vi "main_state.vi"() -> ()   [LabVIEW 2012]
uses:
  machine_type.ctl
  <vilib>/LabVIEW Interface for Arduino/LabVIEW Interface for Arduino.lvlib
  LIFA Ultrasonic Distance LV9/LIFA Ultrasonic Distance.lvlib
  LIFA Ultrasonic Distance LV9/Get Distance/HC-SR04 Get Distance.vi
panel:
  in  "stop":bool
  in  "Plot Color":u32(colorbox)=16715776
  in  "Grid Color":u32(colorbox)
  in  "Visible Section":u16(ring)=8
  in  "Lines/Points":enum16{"Lines", "Points"}(ring)
  out "Polar Plot":picture
  out "Current angle (Degrees)":u8=15
  in  "Speed":u8=1
  in  "Servo 0 Sweep Max Angle":u8=180
  out "Current distance (cm)":dbl
  in  "Signal Pin":u8
  in  "Trigger Pin":u8
  in  "Servo Data Pin":u8=12
  in  "VISA resource":refnum<visa-resource-name>
  in  "Enum":T1
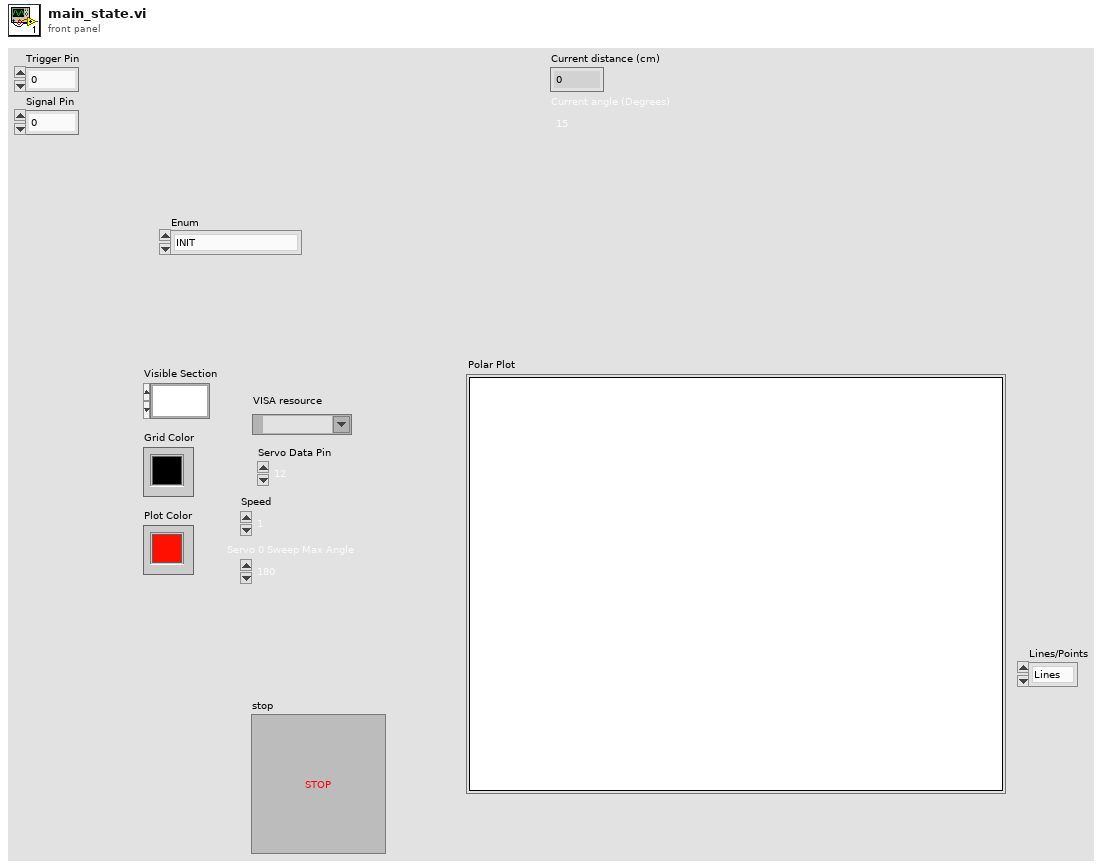
[diagram p1: front panel]
types:
  T1 = typedef "machine_type.ctl" = enum16{"INIT", "MEASURE_DIST", "MOVE_SERVO", "CLOSE", "PLOT_DATA", "ERROR"}
  T2 = typedef "LabVIEW Interface for Arduino.lvlib/Arduino Resource.ctl" = cluster{"VISA resource":refnum<visa-resource-name>, "Board Type":T3, "Connection Type":enum8{"USB / Serial"}, "Bytes Per Packet (15)":u8}
  T3 = typedef "LabVIEW Interface for Arduino.lvlib/Board Type.ctl" = enum16{"Uno", "Dimuelanove w/Atmega 328", "Mega 2560"}
  T4 = cluster{"maximum":dbl, "minimum":dbl, "clip to min":bool, "log?(F)":bool, "grid color":u32, "plot color":u32, "format and precision":cluster{"format":enum8{"Decimal", "Scientific", "Engineering", "Binary", "Octal", "Hex"}, "precision":u8}, "visible section":u16}
  T5 = typedef "LVBoundsTypeDef.ctl" = cluster{"Width":u32, "Height":u32}
  T6 = cluster{"Distance (cm)":dbl, "Angle (Degrees)":u8}
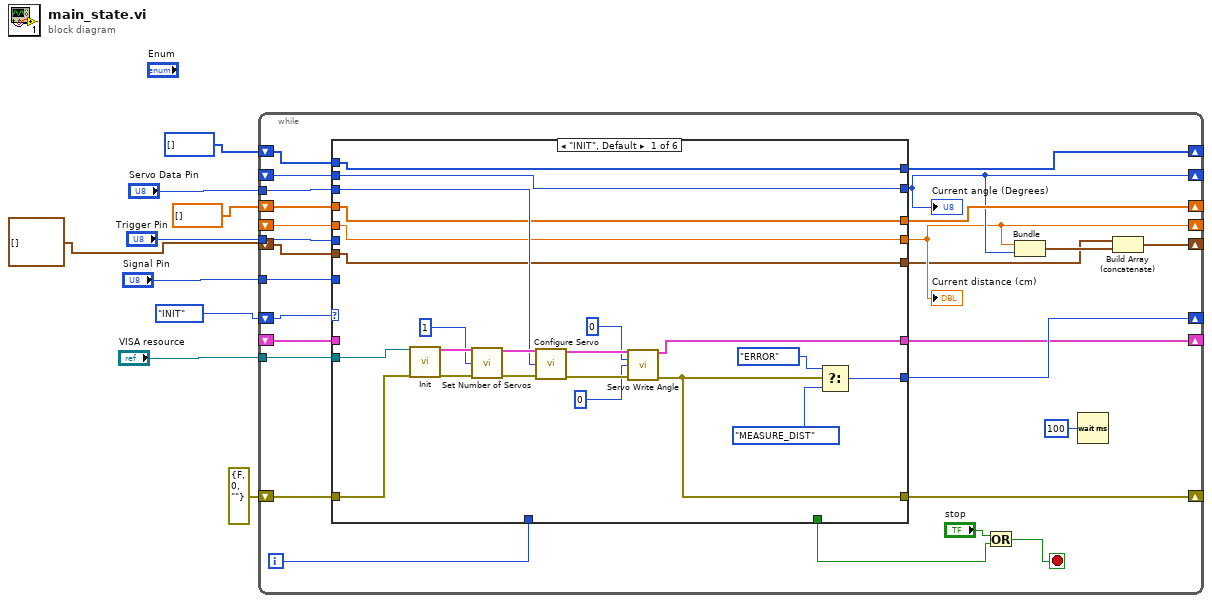
[diagram p0: block diagram]
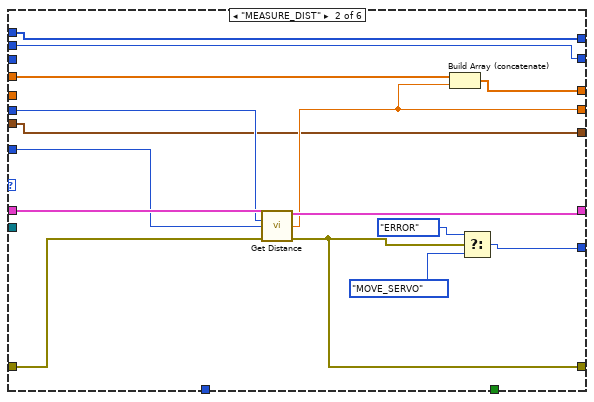
[diagram p2: hidden frame]
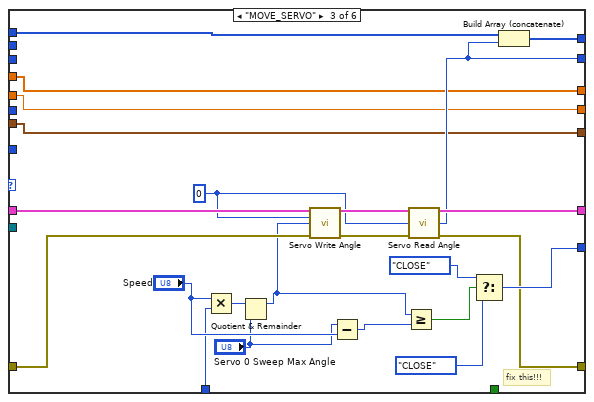
[diagram p3: hidden frame]
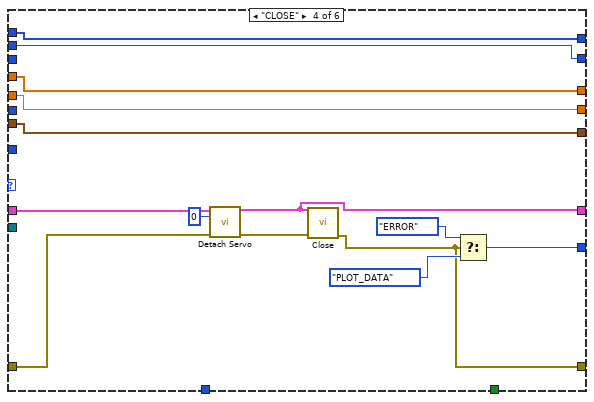
[diagram p4: hidden frame]
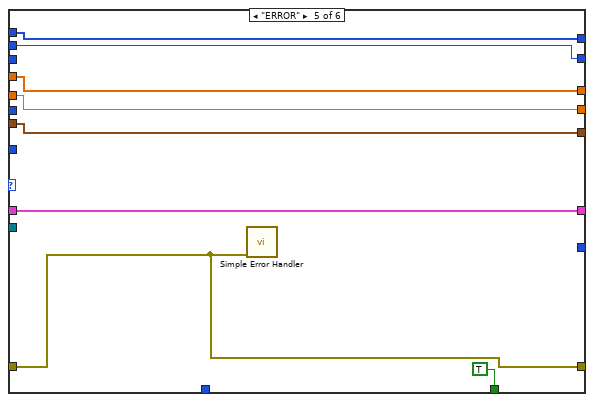
[diagram p5: hidden frame]
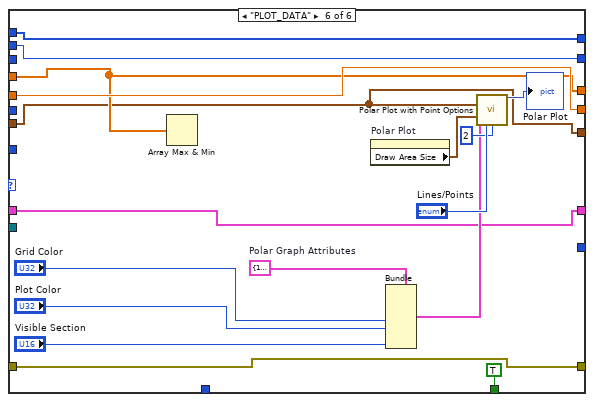
[diagram p6: hidden frame]
diagram:
  n1 = while {
    tunnel: "VISA resource" -> [w36]
    tunnel: "Servo Data Pin" -> [w35]
    shift-right: [w34] -> _
    shift-left: machine_type."INIT" ("Enum 2") -> [w10]
    shift-right: [w33] -> _
    shift-left: errorcluster {"status"=FALSE, "code"=0, "source"=""} ("error out") -> [w32]
    shift-right: [w31] -> _
    shift-left: _ -> [w30]
    tunnel: "Trigger Pin" -> [w29]
    tunnel: "Signal Pin" -> [w28]
    shift-right: [w20] -> _
    shift-left: _ -> [w15]
    shift-right: [w21] -> _
    shift-left: _ -> [w26]
    shift-right: [w24] -> _
    shift-left: dbl[] [] -> [w25]
    shift-right: [w22] -> _
    shift-left: u8[] [] -> [w23]
    shift-right: [w16] -> _
    shift-left: cluster{"magnitude":dbl, "phase":dbl}[] [] ("data array [mag, phase (deg)]") -> [w18]
    i -> [w27]
    stop <- w11 stop-if-true
    n2 = case shown="\"INIT\", Default" w10 {
      tunnel: w36 -> [w49 _ _ _ _ _]
      tunnel: w35 -> [w48 _ _ _ _ _]
      tunnel: [w45 w66 w81 w105 _ _] -> w34
      tunnel: [w44 w65 w80 w99 w113 w119] -> w33
      tunnel: w32 -> [w43 w70 w93 w109 w113 w119]
      tunnel: [w42 w69 w85 w102 w116 w124] -> w31
      tunnel: w30 -> [_ w73 w94 w110 w116 w124]
      tunnel: w29 -> [_ w72 _ _ _ _]
      tunnel: w28 -> [_ w71 _ _ _ _]
      tunnel: [w40 w63 w76 w101 w115 w125] -> w20
      tunnel: w27 -> [_ _ w88 _ _ _]
      tunnel: [w41 w60 w78 w103 w117 w120] -> w21
      tunnel: [_ _ _ _ TRUE TRUE] -> w12
      tunnel: w26 -> [w41 w60 _ w103 w117 w120]
      tunnel: w25 -> [w39 w64 w74 w100 w114 w123]
      tunnel: [w39 w62 w74 w100 w114 w123] -> w24
      tunnel: w23 -> [w38 w59 w79 w98 w112 w121]
      tunnel: [w38 w59 w77 w98 w112 w121] -> w22
      tunnel: w18 -> [w37 w61 w75 w97 w111 w122]
      tunnel: [w37 w61 w75 w97 w111 w122] -> w17
      tunnel: w15 -> [w40 _ w76 w101 w115 w125]
      frame "INIT", Default {
        n3 = call <vilib>:"Init.vi"("VISA resource"=w49, "error in"=w43) -> ("Arduino Resource"=w53:T2, "error out"=w54:errorcluster)  [unwired: 16 in]
        n4 = call <vilib>:"Set Number of Servos.vi"("Arduino Resource"=w53, "Number Of Servos (1)"=u8 1, "error in"=w54) -> ("Arduino Resource"=w55:T2, "error out"=w56:errorcluster)  [unwired: 11 in]
        n5 = call <vilib>:"Configure Servo.vi"("Arduino Resource"=w55, "DIO Pin (2)"=w48, "error in"=w56) -> ("Arduino Resource"=w57:T2, "error out"=w58:errorcluster)  [unwired: 11 in]
        n6 = call <vilib>:"Servo Write Angle.vi"("Arduino Resource"=w57, "Servo Number"=u8 0, "Angle (Degrees)"=u8 0, "error in"=w58) -> ("Arduino Resource"=w42:T2, "error out"=w44:errorcluster)  [unwired: 10 in]
        n7 = Select(t=machine_type."ERROR" ("Enum 2"), s=w44, f=machine_type."MEASURE_DIST" ("Enum 2")) -> (s? t:f=w45:T1)
      }
      frame "MEASURE_DIST" {
        n8 = call-poly "Get Distance.vi"("Arduino Resource"=w73, "Trigger Pin"=w72, "Signal Pin"=w71, "error in (no error)"=w70) -> ("Arduino Resource"=w69:T2, "Distance (cm)"=w63:dbl, "error out"=w65:errorcluster)  [unwired: 9 in]
        n9 = Build Array (concatenate)(w64, w63) -> (w62:dbl[])
        n10 = Select(t=machine_type."ERROR" ("Enum 2"), s=w65, f=machine_type."MOVE_SERVO" ("Enum 2")) -> (s? t:f=w66:T1)
      }
      frame "MOVE_SERVO" {
        w87 = u8 0 ("Servo Number")
        # "fix this!!!"
        n11 = Multiply(x="Speed", y=w88) -> (x*y=w89:i32)
        n12 = Quotient & Remainder(x=w89, y="Servo 0 Sweep Max Angle") -> (x-y*floor(x/y)=w86:i32)  [unwired: 1 out]
        n13 = call <vilib>:"Servo Write Angle.vi"("Arduino Resource"=w94, "Servo Number"=w87, "Angle (Degrees)"=w86, "error in"=w93) -> ("Arduino Resource"=w96:T2, "error out"=w95:errorcluster)  [unwired: 10 in]
        n14 = Subtract(x="Servo 0 Sweep Max Angle", y="Speed") -> (x-y=w92:u8)
        n15 = Greater Or Equal?(x=w86, y=w92) -> (x >= y?=w84:bool)
        n16 = call <vilib>:"Servo Read Angle.vi"("Arduino Resource"=w96, "Servo Number"=w87, "error in"=w95) -> ("Arduino Resource"=w85:T2, "Angle (Degrees)"=w78:u8, "error out"=w80:errorcluster)  [unwired: 10 in]
        n17 = Select(t=machine_type."CLOSE" ("Enum 2"), s=w84, f=machine_type."CLOSE" ("Enum 2")) -> (s? t:f=w81:T1)
        n18 = Build Array (concatenate)(w79, w78) -> (w77:u8[])
      }
      frame "CLOSE" {
        n19 = call <vilib>:"Detach Servo.vi"("Arduino Resource"=w110, "Servo Number"=u8 0, "error in"=w109) -> ("Arduino Resource"=w102:T2, "error out"=w108:errorcluster)  [unwired: 11 in]
        n20 = call <vilib>:"Close.vi"("Arduino Resource"=w102, "error in"=w108) -> ("error out"=w99:errorcluster)  [unwired: 13 in]
        n21 = Select(t=machine_type."ERROR" ("Enum 2"), s=w99, f=machine_type."PLOT_DATA" ("Enum 2")) -> (s? t:f=w105:T1)
      }
      frame "ERROR" {
        n22 = call <vilib>:"Simple Error Handler.vi"("error in (no error)"=w113) -> ()  [unwired: 4 in, 5 out]
      }
      frame "PLOT_DATA" {
        w127 = T4 {"maximum"=1.0, "minimum"=0.0, "clip to min"=FALSE, "log?(F)"=FALSE, "grid color"=6710886, "plot color"=65280, "format and precision"={"format"=enum."Decimal", "precision"=1}, "visible section"=0}  # Polar Graph Attributes
        n23 = Array Max & Min(array=w123) -> ()  [unwired: 4 out]
        n24 = property on="Polar Plot" class="Pict"() -> ("Draw Area Size"=w133:T5)  [unwired: 2 in, 2 out]
        n25 = Bundle(cluster=w127, "grid color"="Grid Color", "plot color"="Plot Color", "visible section"="Visible Section") -> (w126:T4)  [unwired: 5 in]
        n26 = call <vilib>:"Polar Plot with Point Options.vi"("data array [mag, phase (deg)]"=w122, "dimensions (w,h)"=w133, "polar attributes"=w126, "Lines/Points"="Lines/Points", "Size"=u16 2) -> ("new picture"=→"Polar Plot":picture)  [unwired: 10 in]
      }
    }
    "Current distance (cm)" <- w20
    "Current angle (Degrees)" <- w21
    n27 = Or(x="stop", y=w12) -> (x .or. y?=w11:bool)
    n28 = Bundle("Distance (cm)"=w20, "Angle (Degrees)"=w21) -> (w19:T6)  [unwired: 1 in]
    n29 = Wait (ms)(milliseconds to wait=u32 100) -> ()  [unwired: 1 out]
    n30 = Build Array (concatenate)(w17, w19) -> (w16:cluster{"Distance (cm)":dbl, "phase":dbl}[])
  }
